vi "Unpack Menu Activation.vi"(11 "MenuActivationMsg in":refnum<class "MenuActivationMsg.lvclass">) -> (0 "Time":u32, 1 "App Item?":bool, 2 "VIRef":refnum<vi>, 3 "MenuRef":refnum<k9>)   [LabVIEW 2020, in "ActorEvents.lvlib" / "MenuActivationMsg.lvclass"]
uses:
  <vilib>/gpm_packages/@cs/mva-viewable/Source/ActorEvents/IEventAggregator Messages/Menu Activation Msg/MenuActivationMsg.lvclass
  <vilib>/gpm_packages/@cs/mva-viewable/Source/ActorEvents/IEventAggregator Messages/Menu Activation Msg/MenuActivationMsg.lvclass/MenuActivationMsg.ctl
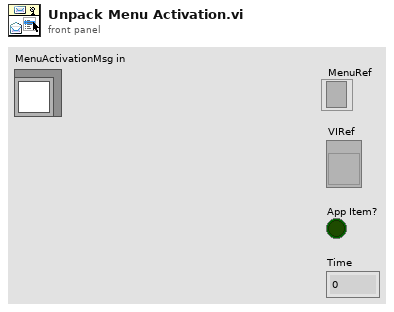
[diagram p1: front panel]
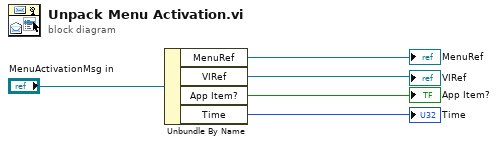
[diagram p0: block diagram]
diagram:
  n1 = Unbundle By Name("MenuActivationMsg in") -> ("MenuRef"=→"MenuRef":refnum<k9>, "VIRef"=→"VIRef":refnum<vi>, "App Item?"=→"App Item?":bool, "Time"=→"Time":u32)
